vi "RAW Data FGV.vi"(7 "Actions":T1=enum."Clear", 8 "error in (no error)":errorcluster, 11 "Handle":u64) -> (0 "error out":errorcluster, 3 "Raw Data":refnum<class "Scan Pattern.lvclass">)   [LabVIEW 2018]
uses:
  General/Controls/FGV Actions.ctl
  SpectralRadar/LabVIEW/2012/user.lib/SpectralRadar.llb/Scan Pattern.lvclass
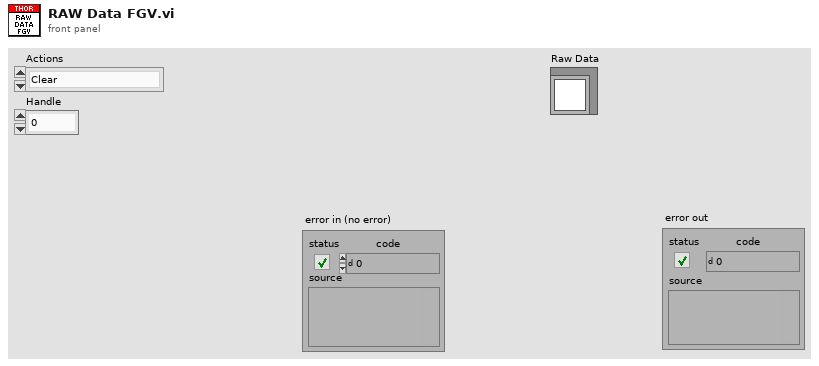
[diagram p1: front panel]
types:
  T1 = typedef "FGV Actions.ctl" = enum16{"Init", "Set", "Get", "Clear"}
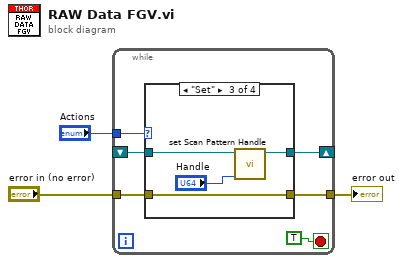
[diagram p0: block diagram]
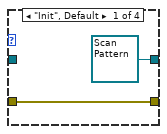
[diagram p2: hidden frame]
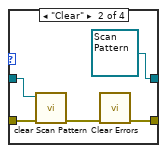
[diagram p3: hidden frame]
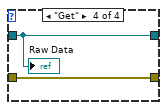
[diagram p4: hidden frame]
diagram:
  n1 = while {
    shift-right: [w9] -> _
    shift-left: _ -> [w8]
    tunnel: "Actions" -> [w7]
    tunnel: "error in (no error)" -> [w6]
    tunnel: [w5] -> w1
    stop <- TRUE stop-if-true
    n2 = case shown="\"Set\"" w7 {
      tunnel: [refnum<class "Scan Pattern.lvclass"> refnum ("Scan Pattern") refnum<class "Scan Pattern.lvclass"> refnum ("Scan Pattern") w20 w22] -> w9
      tunnel: w8 -> [_ w14 w18 w22]
      tunnel: w6 -> [w10 w13 w17 w21]
      tunnel: [w10 w12 w17 w21] -> w5
      frame "Init", Default {
      }
      frame "Clear" {
        n3 = call "clear Scan Pattern.vi"("error in (no error)"=w13, "Scan Pattern in"=w14) -> ("error out"=w15:errorcluster)  [unwired: 5 in]
        n4 = call <vilib>:"Clear Errors.vi"("error in (no error)"=w15) -> ("error out"=w12:errorcluster)  [unwired: 5 in, 1 out]
      }
      frame "Set" {
        n5 = call "set Scan Pattern Handle.vi"("Handle"="Handle", "Scan Pattern"=w18) -> ("Scan Pattern"=w20:refnum<class "Scan Pattern.lvclass">)  [unwired: 5 in]
      }
      frame "Get" {
        "Raw Data" <- w22
      }
    }
  }
  "error out" <- w1
